vi "Para_Script.vi"(11 "TS Parameter":T1={"ProfitCenterCode"="", "LineCode"="", "WorkOrderNumber"="", "Model"="", "Model_with_Prefix"="", "VendorCode"="", "SetParameterDateCode"="", "PokaYoke"=0, "Target"=1, "Live_DateCode"="", "CustomerPartNumber"="", "Hose_Type"="", "sBarcode"=FALSE, "FCA"=0, "Ent_Stamp"=timestamp(0 s since 1904-01-01), "STS_CD"=0.0} {"FCA" format="%01d"; "Target" min=1 max=100000; "PokaYoke" min=0 max=1}) -> (0 "Update Script":string, 3 "iNSERT Script":string)   [LabVIEW 2020]
uses:
  Controls/TS_Parameter_V2.ctl
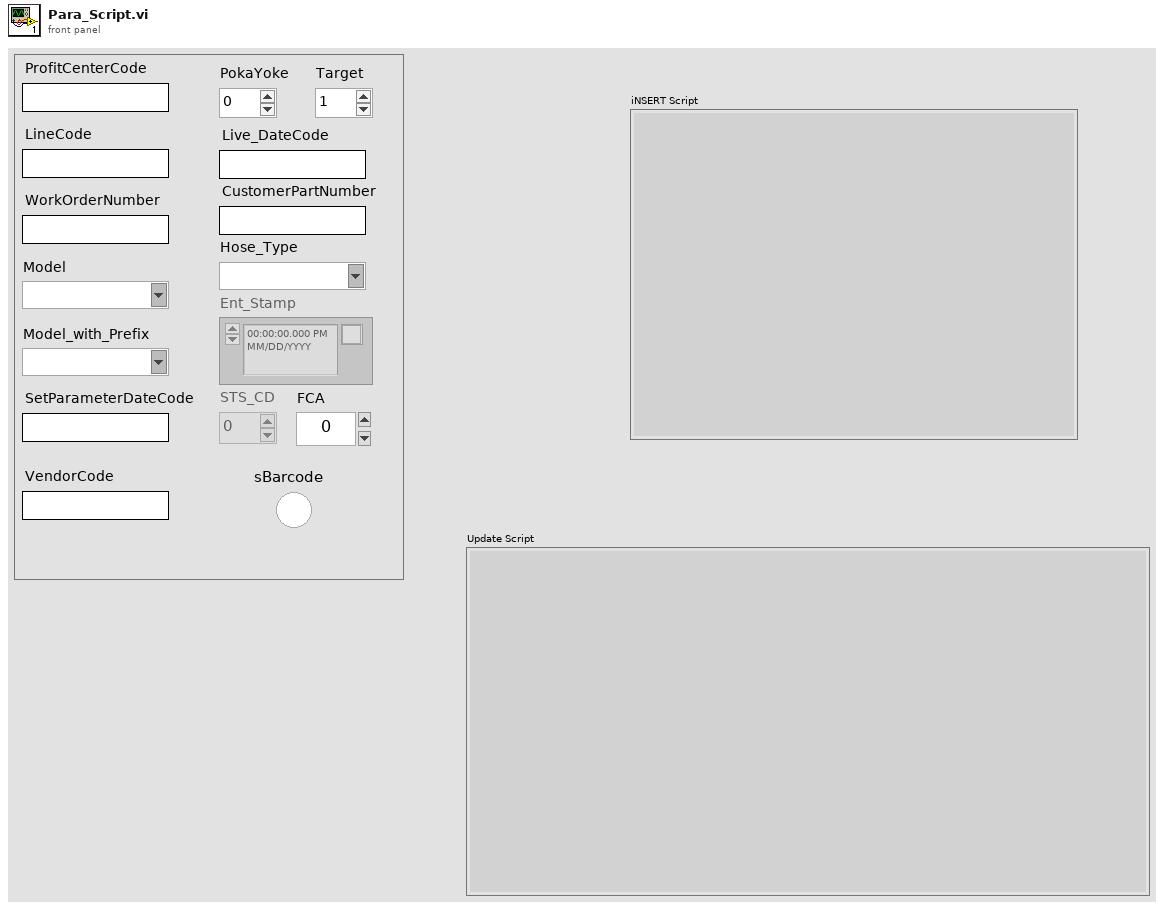
[diagram p1: front panel]
types:
  T1 = typedef "TS_Parameter_V2.ctl" = cluster{"ProfitCenterCode":string, "LineCode":string, "WorkOrderNumber":string, "Model":string, "Model_with_Prefix":string, "VendorCode":string, "SetParameterDateCode":string, "PokaYoke":i32, "Target":i32, "Live_DateCode":string, "CustomerPartNumber":string, "Hose_Type":string, "sBarcode":bool, "FCA":i32, "Ent_Stamp":timestamp, "STS_CD":dbl}
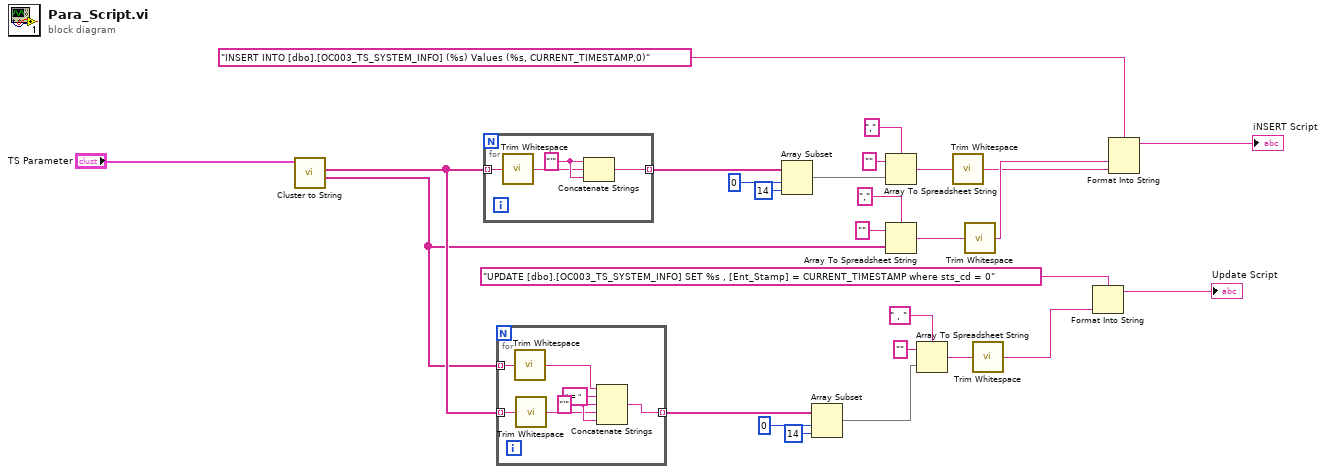
[diagram p0: block diagram]
diagram:
  n1 = call <userlib>:"Cluster to String.vi"("Variant In"="TS Parameter") -> ("Format String Name"=w12:string[], "Format String Array"=w13:string[])  [unwired: 7 in, 2 out]
  n2 = for {
    tunnel: w13 -> [w31] mode=indexing
    tunnel: [w29] -> w14 mode=indexing
    w30 = "'" ("string")
    n3 = call <vilib>:"Trim Whitespace.vi"("string"=w31) -> ("trimmed string"=w28:string)  [unwired: 1 in]
    n4 = Concatenate Strings(w30, w28, w30) -> (w29:string)
  }
  n5 = for {
    tunnel: [w37] -> w9 mode=indexing
    tunnel: w13 -> [w35] mode=indexing
    tunnel: w12 -> [w34] mode=indexing
    w38 = "'" ("string")
    n6 = call <vilib>:"Trim Whitespace.vi"("string"=w34) -> ("trimmed string"=w33:string)  [unwired: 1 in]
    n7 = call <vilib>:"Trim Whitespace.vi"("string"=w35) -> ("trimmed string"=w36:string)  [unwired: 1 in]
    n8 = Concatenate Strings(w33, " = " ("string"), w38, w36, w38) -> (w37:string)
  }
  n9 = Array Subset(array=w14, index=0, length=14) -> (w21:string[])
  n10 = Array Subset(array=w9, index=0, length=14) -> (w6:string[])
  n11 = Array To Spreadsheet String(delimiter (Tab)=",", array=w21, 3:"" ("format string")) -> (spreadsheet string=w17:string)
  n12 = Array To Spreadsheet String(delimiter (Tab)=",", array=w12, 3:"" ("format string")) -> (spreadsheet string=w25:string)
  n13 = Array To Spreadsheet String(delimiter (Tab)=" , ", array=w6, 3:"" ("format string")) -> (spreadsheet string=w5:string)
  n14 = call <vilib>:"Trim Whitespace.vi"("string"=w17) -> ("trimmed string"=w15:string)  [unwired: 1 in]
  n15 = call <vilib>:"Trim Whitespace.vi"("string"=w25) -> ("trimmed string"=w18:string)  [unwired: 1 in]
  n16 = call <vilib>:"Trim Whitespace.vi"("string"=w5) -> ("trimmed string"=w2:string)  [unwired: 1 in]
  n17 = Format Into String(format string="UPDATE [dbo].[OC003_TS_SYSTEM_INFO] SET %s , [Ent_Stamp] = CURRENT_TIMESTAMP where sts_cd = 0", w2) -> (resulting string=→"Update Script":string)  [unwired: 2 in, 1 out]
  n18 = Format Into String(format string="INSERT INTO [dbo].[OC003_TS_SYSTEM_INFO] (%s) Values (%s, CURRENT_TIMESTAMP,0)", w18, w15) -> (resulting string=→"iNSERT Script":string)  [unwired: 2 in, 1 out]
